vi "Curtin1_ReadSaveTemplate.vi"(6 "Task":enum16{"Save", "Read", "List"}(ring), 9 "Template":string="favorites.txt", 11 "Settings":T1={"Name of test"="ScratchPad", "Date"=timestamp(0 s since 1904-01-01), "Location"="Home", "Template"="Simple", "Soundcard"="OCTA-CAPTURE", "resolution"=32, "Sampling rate"=48000, "Ch1 Gain "=25.0, "Ch2 Gain"=10.0, "Sample time (s)"=0.3, "Pre-trigger (s)"=0.001, "Hammer Threshold"=10.0, "Positions"=12, "Taps/Position"=5, "Set Names"="H,V", "Freq resolution"=1.0, "Hammer cutoff"=0.025, "Mic cutoff"=0.25, "Double bounce "=10.0, "Hammer Cal"=10.0, "dB Offset"=0.0, "Accel Cal"=10.0, "Vibrometer Cal"=0.0, "Mic Cal"=0.0, "Output"=2, "Voltage Cal"=1.0, "Vibrometer Port"="ASRL27::INSTR", "Range"=4, "High Pass"=2, "Bandwidth"=4, "X Range"=[], "Y Range"=[], "dB Spread"=0.0, "Trigger"=0, "Ch_1"=25, "Ch_2"=25, "flip?"=FALSE, "60Hz"=FALSE, "Time offset"=0.0, "Piezo Cal"=1.0, "Default Notes"="", "Tom"=FALSE} {"Ch_2" min=1 step=1; "Ch_1" min=1 max=100 step=1; "Trigger" items=["Hammer (force)", "Self-tap", "Spacebar"]; "Bandwidth" items=["1 kHz"=1, "5 kHz"=5, "10 kHz"=10, "25 kHz"=25, "50 kHz"=50, "100 kHz"=100]; "High Pass" items=["Off", "13 Hz", "104 Hz"]; "Range" items=["10 mm/s"=1, "20 mm/s"=2, "50 mm/s"=5, "100 mm/s"=10, "200 mm/s"=20, "500 mm/s"=50, "1 m/s"=100, "2 m/s"=200]; "Output" items=["Accelerometer", "Speed (from acceleration)", "Microphone", "Vibrometer", "Piezo"]; "Voltage Cal" format="%#_13g"; "Ch2 Gain" format="%#_13g"; "Ch1 Gain" format="%#_13g"; "Double bounce" min=0.0; "Mic cutoff" min=0.0 format="%#_4g"; "Hammer cutoff" min=0.0 format="%#_4g"; "Freq resolution" min=0.0; "Pre-trigger (s)" format="%#_13g"; "Date" format="%<%H:%M\n%d/%m/%y>T"; "resolution" items=["16 bit"=16, "24 bit"=24, "32 bit"=32]; "Sampling rate" items=["22050 samp/s"=22050, "44100 samp/s"=44100, "48000 samp/s"=48000]}) -> (0 "error out":errorcluster, 1 "String":string, 2 "List":string[](array[string]), 3 "Settings out":T1={"Name of test"="", "Date"=timestamp(0 s since 1904-01-01), "Location"="", "Template"="", "Soundcard"="", "resolution"=32, "Sampling rate"=48000, "Ch1 Gain "=25.0, "Ch2 Gain"=10.0, "Sample time (s)"=0.3, "Pre-trigger (s)"=0.01, "Hammer Threshold"=10.0, "Positions"=12, "Taps/Position"=5, "Set Names"="", "Freq resolution"=10.0, "Hammer cutoff"=0.0, "Mic cutoff"=0.0, "Double bounce "=0.0, "Hammer Cal"=10.0, "dB Offset"=0.0, "Accel Cal"=10.0, "Vibrometer Cal"=0.0, "Mic Cal"=0.0, "Output"=2, "Voltage Cal"=1.0, "Vibrometer Port"="ASRL27::INSTR", "Range"=4, "High Pass"=2, "Bandwidth"=4, "X Range"=[], "Y Range"=[], "dB Spread"=0.0, "Trigger"=0, "Ch_1"=25, "Ch_2"=25, "flip?"=FALSE, "60Hz"=FALSE, "Time offset"=0.0, "Piezo Cal"=1.0, "Default Notes"="", "Tom"=FALSE} {"Ch_2" min=1 step=1; "Ch_1" min=1 max=100 step=1; "Trigger" items=["Hammer (force)", "Self-tap", "Spacebar"]; "Bandwidth" items=["1 kHz"=1, "5 kHz"=5, "10 kHz"=10, "25 kHz"=25, "50 kHz"=50, "100 kHz"=100]; "High Pass" items=["Off", "13 Hz", "104 Hz"]; "Range" items=["10 mm/s"=1, "20 mm/s"=2, "50 mm/s"=5, "100 mm/s"=10, "200 mm/s"=20, "500 mm/s"=50, "1 m/s"=100, "2 m/s"=200]; "Output" items=["Accelerometer", "Speed (from acceleration)", "Microphone", "Vibrometer", "Piezo"]; "Voltage Cal" format="%#_13g"; "Ch2 Gain" format="%#_13g"; "Ch1 Gain" format="%#_13g"; "Double bounce" min=0.0; "Mic cutoff" min=0.0 format="%#_4g"; "Hammer cutoff" min=0.0 format="%#_4g"; "Freq resolution" min=0.0; "Pre-trigger (s)" format="%#_13g"; "Date" format="%<%H:%M\n%d/%m/%y>T"; "resolution" items=["16 bit"=16, "24 bit"=24, "32 bit"=32]; "Sampling rate" items=["22050 samp/s"=22050, "44100 samp/s"=44100, "48000 samp/s"=48000]})   [LabVIEW 2022 SP3]
uses:
  Mic/Mic_Global.vi
  PreferencesControl.ctl
panel:
  # "Hz"
  # "dB"
  # "dB"
  # "sec"
  # "sec"
  # "mV/Pa"
  # "mV/m/s2"
  # "mV/mm/s"
  # "V/N"
  # "sec"
  # "sec"
  # "mV/N"
  # "a.u."
  # "a.u."
  # "sec"
  # "Hz"
  # "dB"
  # "dB"
  # "sec"
  # "sec"
  # "mV/Pa"
  # "mV/m/s2"
  # "mV/mm/s"
  # "V/N"
  # "sec"
  # "sec"
  # "mV/N"
  # "a.u."
  # "a.u."
  # "sec"
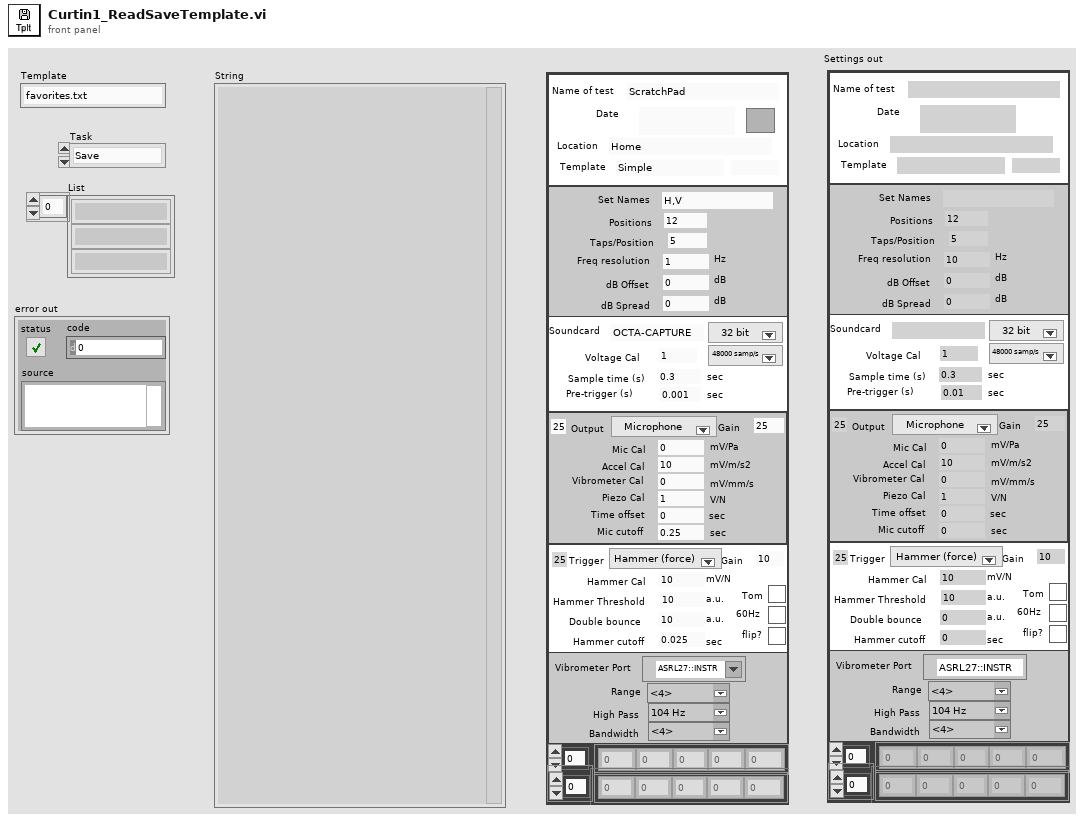
[diagram p1: front panel]
types:
  T1 = typedef "PreferencesControl.ctl" = cluster{"Name of test":string, "Date":timestamp, "Location":string, "Template":string, "Soundcard":string, "resolution":u16, "Sampling rate":u16, "Ch1 Gain ":dbl, "Ch2 Gain":dbl, "Sample time (s)":dbl, "Pre-trigger (s)":dbl, "Hammer Threshold":dbl, "Positions":i16, "Taps/Position":i16, "Set Names":string, "Freq resolution":dbl, "Hammer cutoff":dbl, "Mic cutoff":dbl, "Double bounce ":dbl, "Hammer Cal":dbl, "dB Offset":dbl, "Accel Cal":dbl, "Vibrometer Cal":dbl, "Mic Cal":dbl, "Output":u16, "Voltage Cal":dbl, "Vibrometer Port":refnum<visa-resource-name>, "Range":u16, "High Pass":u16, "Bandwidth":u16, "X Range":cluster{"Minimum":dbl, "Maximum":dbl, "Increment":dbl, "Minor Increment":dbl, "Start":dbl}[], "Y Range":cluster{"Minimum":dbl, "Maximum":dbl, "Increment":dbl, "Minor Increment":dbl, "Start":dbl}[], "dB Spread":dbl, "Trigger":u16, "Ch_1":u8, "Ch_2":u8, "flip?":bool, "60Hz":bool, "Time offset":dbl, "Piezo Cal":dbl, "Default Notes":string, "Tom":bool}
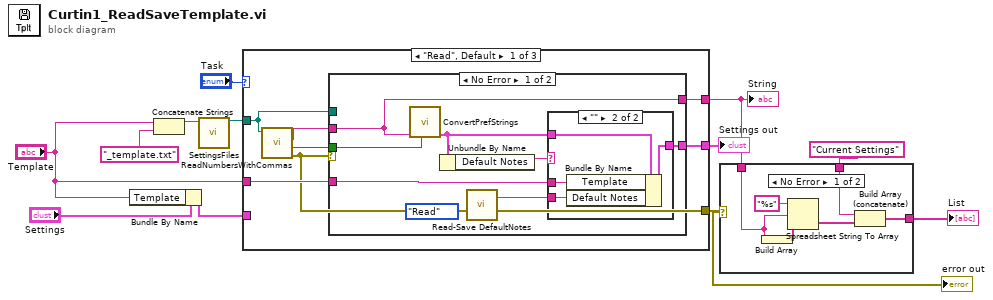
[diagram p0: block diagram]
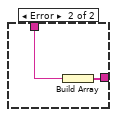
[diagram p2: hidden frame]
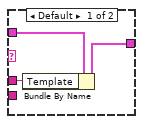
[diagram p3: hidden frame]
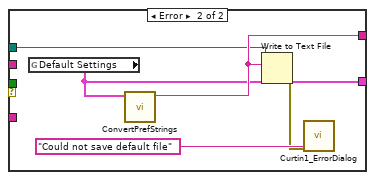
[diagram p4: hidden frame]
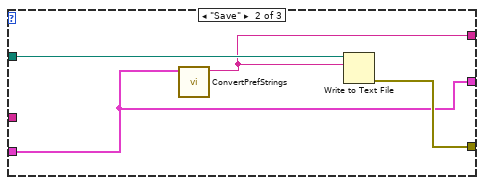
[diagram p5: hidden frame]
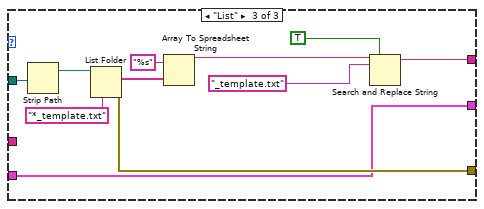
[diagram p6: hidden frame]
diagram:
  n1 = Bundle By Name(cluster="Settings", "Template"="Template") -> (w4:T1)
  n2 = Concatenate Strings("Template", "_template.txt" ("string")) -> (w2:string)
  n3 = call "SettingsFiles.vi"("settings file name"=w2) -> ("file path"=w1:path)  [unwired: 9 in, 1 out]
  n4 = case shown="\"Read\", Default" "Task" {
    tunnel: w1 -> [w16 w43 w54]
    tunnel: [w14 w42 w45] -> w7
    tunnel: [w19 w41 w49] -> w9
    tunnel: [w18 w40 w44] -> w6
    tunnel: w4 -> [_ w40 w44]
    tunnel: "Template" -> [w17 _ _]
    frame "Read", Default {
      n5 = call "ReadNumbersWithCommas.vi"("file (use dialog)"=w16) -> ("error out"=w14:errorcluster, "comma?"=w13:bool, "text"=w15:string)  [unwired: 7 in, 1 out]
      n6 = case shown="No Error" w14 {
        tunnel: w15 -> [w27 _]
        tunnel: [w27 w39] -> w19
        tunnel: [w25 w38] -> w18
        tunnel: w16 -> [_ w37]
        tunnel: w17 -> [w26 _]
        tunnel: w13 -> [w24 _]
        frame No Error {
          n7 = call "ConvertPrefStrings.vi"("Comma?"=w24, "String In"=w27) -> ("Settings"=w23:T1)  [unwired: 8 in, 1 out]
          n8 = Unbundle By Name(w23) -> ("Default Notes"=w22:string)
          n9 = call "Read-Save DefaultNotes.vi"("Task"=enum16{"Save", "Read"}."Read") -> ("Notes Out"=w21:string)  [unwired: 9 in, 1 out]
          n10 = case shown="\"\"" w22 {
            tunnel: w26 -> [w30 w34]
            tunnel: [w29 w32] -> w25
            tunnel: w23 -> [w28 w33]
            tunnel: w21 -> [_ w31]
            frame Default {
              n11 = Bundle By Name(cluster=w28, "Template"=w30) -> (w29:T1)
            }
            frame "" {
              n12 = Bundle By Name(cluster=w33, "Template"=w34, "Default Notes"=w31) -> (w32:T1)
            }
          }
        }
        frame Error {
          n13 = global read "Mic_Global.vi" "Default Settings"() -> (w38:T1)
          n14 = call "ConvertPrefStrings.vi"("Settings"=w38) -> ("String Out"=w39:string)  [unwired: 9 in, 1 out]
          n15 = Write to Text File(file (use dialog)=w37, text=w39) -> (error out=w35:errorcluster)  [unwired: 2 in, 2 out]
          n16 = call "Curtin1_ErrorDialog.vi"("error in (no error)"=w35, "String"="Could not save default file") -> ()  [unwired: 9 in, 1 out]
        }
      }
    }
    frame "Save" {
      n17 = call "ConvertPrefStrings.vi"("Settings"=w40) -> ("String Out"=w41:string)  [unwired: 9 in, 1 out]
      n18 = Write to Text File(file (use dialog)=w43, text=w41) -> (error out=w42:errorcluster)  [unwired: 2 in, 2 out]
    }
    frame "List" {
      n19 = Strip Path(path=w54) -> (stripped path=w53:path)  [unwired: 1 out]
      n20 = List Folder(path=w53, pattern="*_template.txt") -> (filenames=w51:string[], error out=w45:errorcluster)  [unwired: 2 in, 2 out]
      n21 = Array To Spreadsheet String(array=w51, 3:"%s" ("format string")) -> (spreadsheet string=w48:string)  [unwired: 1 in]
      n22 = Search and Replace String(replace all?=TRUE ("replace all? (F)"), input string=w48, search string="_template.txt") -> (result string=w49:string)  [unwired: 5 in, 3 out]
    }
  }
  "String" <- w9
  "Settings out" <- w6
  "error out" <- w7
  n23 = case shown="No Error" w7 {
    tunnel: "Current Settings" ("String") -> [w57 w62]
    tunnel: w9 -> [w56 _]
    tunnel: [w55 w61] -> w8
    frame No Error {
      n24 = Build Array(w56) -> (w60:string[])
      n25 = Spreadsheet String To Array(format string="%s", spreadsheet string=w56, array type (2D Dbl)=w60) -> (array=w58:string[])  [unwired: 1 in]
      n26 = Build Array (concatenate)(w57, w58) -> (w55:string[])
    }
    frame Error {
      n27 = Build Array(w62) -> (w61:string[])
    }
  }
  "List" <- w8
